vi "Get User's Password.vi"(0 "User Manager Model in":refnum<class "User Manager Model.lvclass">, 5 "Username":string, 11 "error in (no error)":errorcluster) -> (4 "User Manager Model out":refnum<class "User Manager Model.lvclass">, 15 "error out":errorcluster)   [LabVIEW 2017, in "User Manager Model.lvlib" / "User Manager Model.lvclass"]
uses:
  User Manager Model.lvclass
  C:/Program Files/National Instruments/LabVIEW 2017/vi.lib/gpm_packages/@cs/mva-core/Source/IModel/IModel/IModel.lvclass
  User Manager Model.lvclass/User Manager Model.ctl
  <vilib>/gpm_packages/@cs/mva-core/Source/IObserver/IObserver/IObserver.lvclass/IObserver.ctl
  <vilib>/gpm_packages/@cs/mva-core/Source/IModel/IModel/IModel.lvclass/IModel.ctl
  <vilib>/gpm_packages/@cs/mva-core/Source/IMediator/PublishRequest/PublishRequest.lvclass/PublishRequest.ctl
  <vilib>/gpm_packages/@cs/mva-core/Source/IMediator/IMediator Messages/Publish Msg/Publish Msg.lvclass/Publish Msg.ctl
  <vilib>/gpm_packages/@cs/actor-framework-messages/Source/RoundTripMessage/RoundTripMessage.lvclass/RoundTripMessage.ctl
  <vilib>/ActorFramework/Message Enqueuer/Message Enqueuer.lvclass/Message Enqueuer.ctl
  <vilib>/gpm_packages/@cs/mva-core/Source/IMediator/IMediator Messages/Publish Msg/Send Pre-Addressed Publish.vi
  <vilib>/gpm_packages/@cs/mva-core/Source/IObserver/IObserver/Read Unique ID.vi
  <vilib>/gpm_packages/@cs/mva-core/Source/IMediator/PublishRequest/Pack Publish Request.vi
  <vilib>/gpm_packages/@cs/actor-framework-messages/Source/RoundTripMessage/Return Round-Trip Message.vi
  <vilib>/ActorFramework/Message Enqueuer/Enqueue.vi
  <vilib>/gpm_packages/@cs/mva-core/Source/IModel/IModel/IModel.lvclass
  C:/Program Files/National Instruments/LabVIEW 2017/vi.lib/gpm_packages/@cs/mva-core/Source/IObserver/IObserver/IObserver.lvclass
  <vilib>/gpm_packages/@cs/mva-core/Source/IMediator/IMediator Messages/Publish Msg/Publish Msg.lvclass
  C:/Program Files/National Instruments/LabVIEW 2017/vi.lib/gpm_packages/@cs/actor-framework-messages/Source/RoundTripMessage/RoundTripMessage.lvclass
  <vilib>/gpm_packages/@cs/actor-framework-messages/Source/RoundTripMessage/RoundTripMessage.lvclass
  C:/Program Files/National Instruments/LabVIEW 2017/vi.lib/ActorFramework/Message/Message.lvclass
  <vilib>/Utility/error.llb/Error Cluster From Error Code.vi
  <vilib>/ActorFramework/Message Priority Queue/Priority Enqueue.vi
  <vilib>/gpm_packages/@cs/mva-core/Source/IMediator/PublishRequest/PublishRequest.lvclass
  <vilib>/gpm_packages/@cs/user-manager/Source/User Configuration Manager Ref/By Ref.lvlib
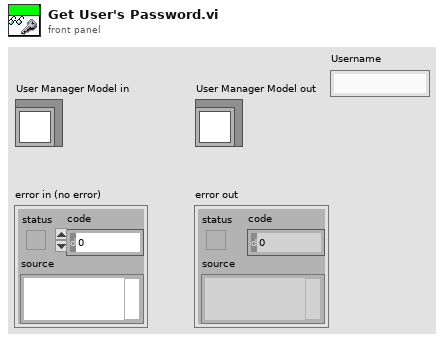
[diagram p1: front panel]
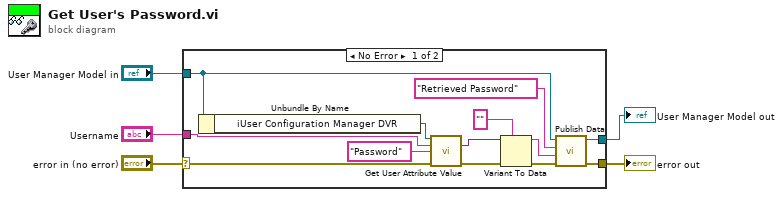
[diagram p0: block diagram]
diagram:
  n1 = case shown="No Error" "error in (no error)" {
    selector: "error in (no error)" -> [w15 w20]
    tunnel: [w14 w20] -> w4
    tunnel: [w16 w19] -> w2
    tunnel: "User Manager Model in" -> [w17 w19]
    tunnel: "Username" -> [w8 _]
    frame No Error {
      n2 = Unbundle By Name(w17) -> ("iUser Configuration Manager DVR"=w18:refnum<data-value>)
      n3 = call <vilib>:"Get User Attribute Value.vi"("iUser Configuration Manager DVR"=w18, "Username"=w8, "Attribute Name"="Password", "error in"=w15) -> ("Attribute Value"=w12:variant, "error out"=w10:errorcluster)  [unwired: 8 in, 2 out]
      n4 = Variant To Data(error in=w10, type="", Variant=w12) -> (data=w11:string, error out=w9:errorcluster)
      n5 = call <vilib>:"Publish Data.vi"("error in (no error)"=w9, "Data to Publish"=w11, "Datum Name"="Retrieved Password", "IModel in"=w17) -> ("error out"=w14:errorcluster, "IModel out"=w16:refnum<class "User Manager Model.lvclass">)  [unwired: 6 in]
    }
    frame Error {
    }
  }
  "error out" <- w4
  "User Manager Model out" <- w2
